vi "calc arcade drive pwm.vi"(3 "error in (no error)":errorcluster, 4 "Y axis value":dbl, 5 "X axis value":dbl) -> (0 "error out":errorcluster, 1 "Right Speed":dbl, 2 "Left Speed":dbl)   [LabVIEW 2013]
uses:
  <vilib>/Rock Robotics/WPI/Solenoid/WPI_SolenoidValue.ctl
  <vilib>/Rock Robotics/SystemInterfaces/NetworkCommunication/NetComm_UsageReport_ResourceType.ctl
  <vilib>/Rock Robotics/WPI/Solenoid/WPI_SolenoidGetEnum.vi
  <vilib>/addons/control/pid/pid.llb/PID (DBL).vi
  <vilib>/Rock Robotics/WPI/RobotDrive/WPI_RobotDriveGetSetRefNum.vi
  <vilib>/addons/control/pid/NI_PID_pid.lvlib
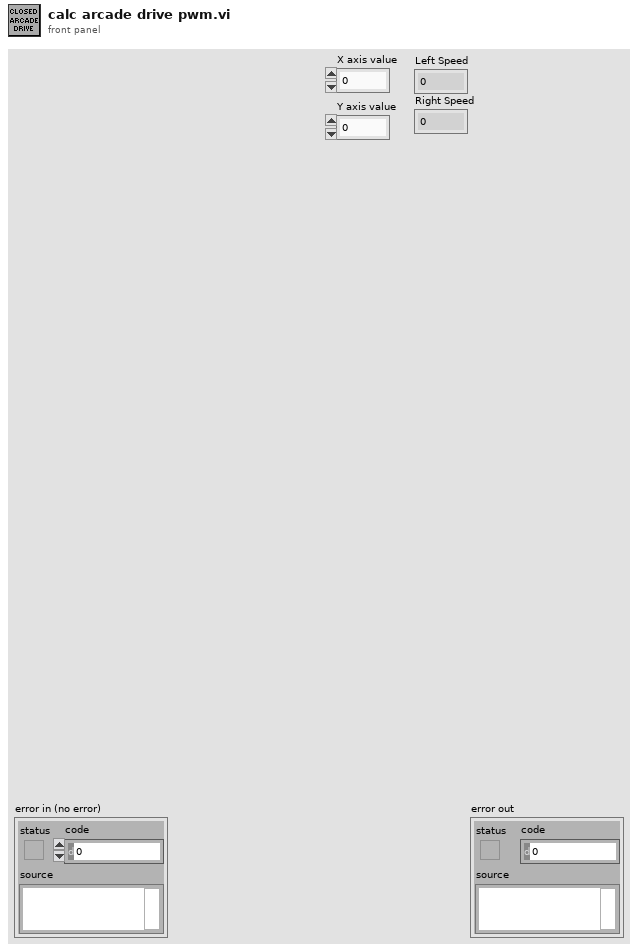
[diagram p1: front panel]
types:
  T1 = cluster{"proportional gain (Kc)":dbl, "integral time (Ti, min)":dbl, "derivative time (Td, min)":dbl}
  T2 = typedef "WPI_SolenoidValue.ctl" = enum16{"Off", "On", "Forward", "Reverse"}
  T3 = typedef "WPI_SolenoidDevRef.ctl" = cluster{"DevStatus":errorcluster, "Solenoid Module":T4, "Forward Solenoid Channel":T5, "Reverse Solenoid Channel":T5}
  T4 = typedef "FPGA_TypedefSolenoidModule.ctl" = enum16{"Solenoid Module 1", "Solenoid Module 2"}
  T5 = typedef "WPI_SolenoidChannel.ctl" = enum8{"Solenoid 1", "Solenoid 2", "Solenoid 3", "Solenoid 4", "Solenoid 5", "Solenoid 6", "Solenoid 7", "Solenoid 8", "Invalid"}
  T6 = typedef "WPI_RobotDriveDevRef.ctl" = cluster{"DevStatus":errorcluster, "Motors[]":T7[], "Square Inputs":bool, "Max Output":dbl, "Isochronous":bool}
  T7 = typedef "WPI_MotorControlDeviceRef.ctl" = cluster{"DeviceStatus":errorcluster, "Type":enum16{"PWM", "CAN"}, "PWM":cluster{"Digital Module":T8, "PWM Channel":T9, "DeadBand":T10}, "CAN":cluster{"Device Number":u8, "Control Mode":T11, "Semaphore":T12, "Max Vout":dbl}, "Invert":bool, "TransformRef":T13, "InvTransformRef":T13}
  T8 = typedef "FPGA_TypedefDigitalModule.ctl" = enum16{"Digital Module 1", "Digital Module 2"}
  T9 = typedef "FPGA_DIOPWMChannel.ctl" = enum8{"PWM 1", "PWM 2", "PWM 3", "PWM 4", "PWM 5", "PWM 6", "PWM 7", "PWM 8", "PWM 9", "PWM 10", "Invalid"}
  T10 = typedef "WPI_PWMDeadband.ctl" = cluster{"Name":string, "maxPositivePwm":i32, "minPositivePwm":i32, "centerPwm":i32, "maxNegativePwm":i32, "minNegativePwm":i32, "angularRange":u16}
  T11 = typedef "WPI_CANJaguar_ControlMode.ctl" = enum8{"Percent VBus", "Current", "Speed", "Position", "Voltage"}
  T12 = typedef "Semaphore RefNum" = refnum<k1>
  T13 = typedef "WPI_PWMTransform_ConPane.ctl" = refnum<vi>
  T14 = typedef "NetComm_UsageReport_ResourceType.ctl" = enum8{"Controller", "Module", "Language", "CANPlugin", "Accelerometer", "ADXL345", "AnalogChannel", "AnalogTrigger", "AnalogTriggerOutput", "CANJaguar", "Compressor", "Counter", "Dashboard", "DigitalInput", "DigitalOutput", "DriverStationCIO", "DriverStationEIO", "DriverStationLCD", "Encoder", "GearTooth", "Gyro", "I2C", "Framework", "Jaguar", "Joystick", "Kinect", "KinectStick", "PIDController", "Preferences", "PWM", "Relay", "RobotDrive", "SerialPort", "Servo", "Solenoid", "SPI", "Task", "Ultrasonic", "Victor", "Button", "Command", "AxisCamera", "PCVideoServer", "SmartDashboard", "Talon", "HiTechnicColorSensor", "HiTechnicAccel", "HiTechnicCompass", "SRF08"}
  T15 = typedef "WPI_EncoderDevRef.ctl" = cluster{"DevStatus":errorcluster, "EncoderIndex":T16, "CounterIndex":T17, "DistancePerCount":dbl, "Decoding Type":T18}
  T16 = typedef "FPGA_EncoderIdx.ctl" = enum8{"Enc 0", "Enc 1", "Enc 2", "Enc 3", "Invalid"}
  T17 = typedef "FPGA_CounterCtrSystemIndex.ctl" = enum8{"Ctr 0", "Ctr 1", "Ctr 2", "Ctr 3", "Ctr 4", "Ctr 5", "Ctr 6", "Ctr 7", "Invalid"}
  T18 = typedef "WPI_EncoderType.ctl" = enum16{"1x", "2x", "4x"}
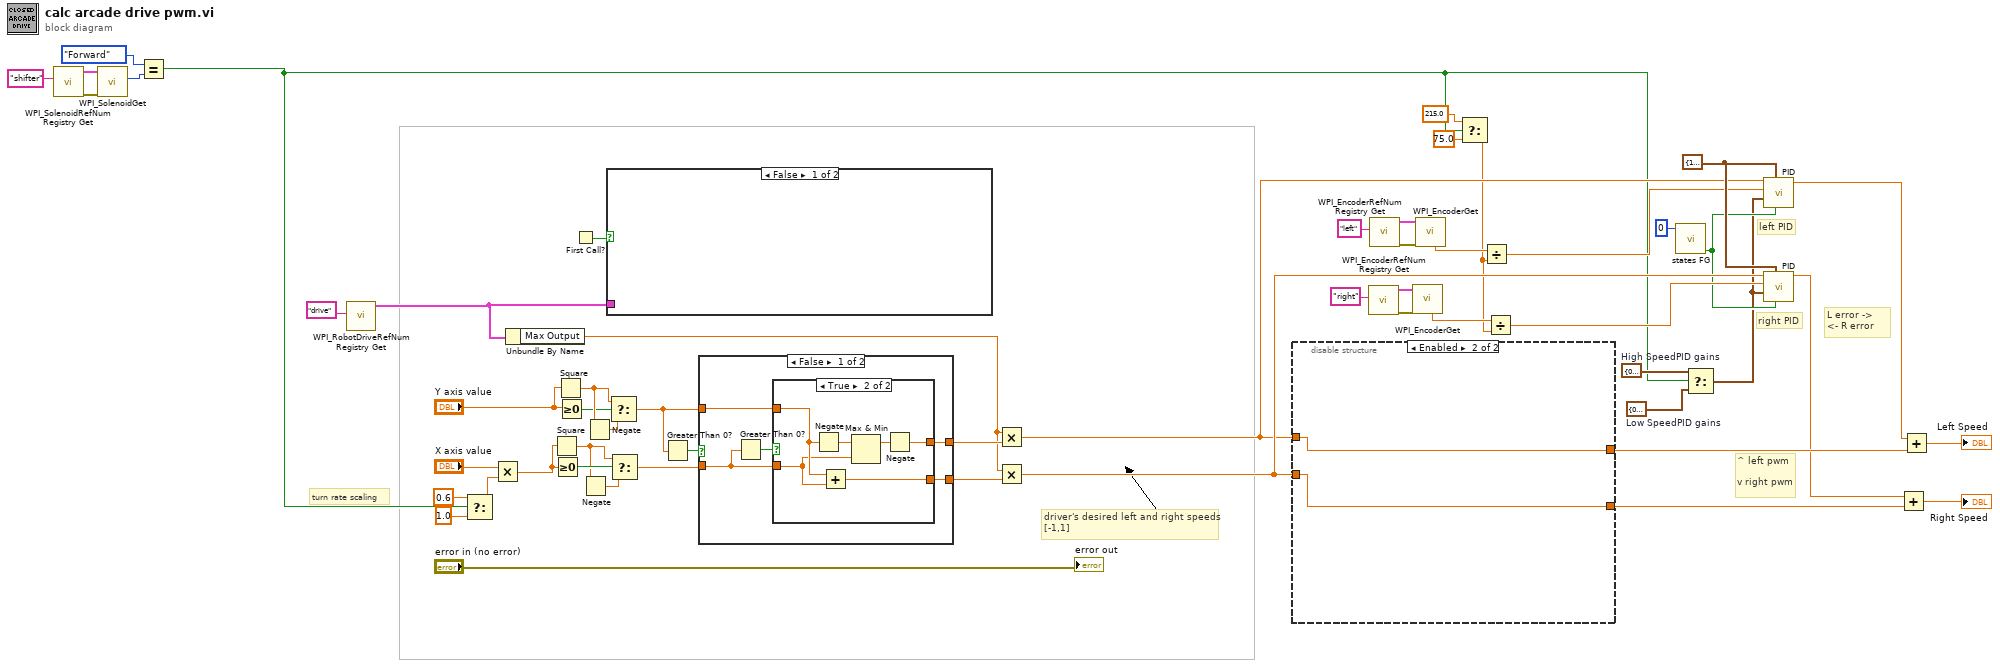
[diagram p0: block diagram]
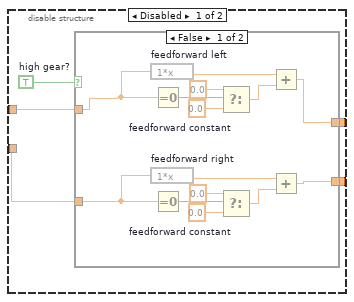
[diagram p2: hidden frame]
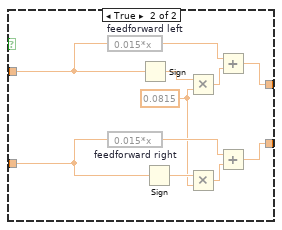
[diagram p3: hidden frame]
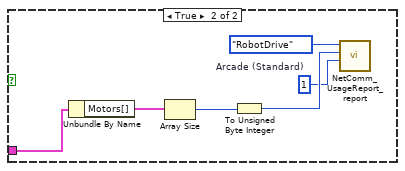
[diagram p4: hidden frame]
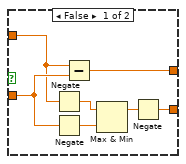
[diagram p5: hidden frame]
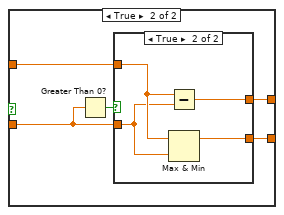
[diagram p6: hidden frame]
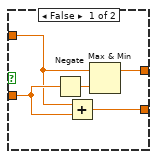
[diagram p7: hidden frame]
diagram:
  w3 = T1 {"proportional gain (Kc)"=0.07, "integral time (Ti, min)"=0.0005, "derivative time (Td, min)"=0.0}  # Low SpeedPID gains
  w4 = T1 {"proportional gain (Kc)"=0.085, "integral time (Ti, min)"=0.0003, "derivative time (Td, min)"=0.0}  # High SpeedPID gains
  w31 = cluster{"output high":dbl, "output low":dbl} {"output high"=1.0, "output low"=-1.0} ("output range")
  # "turn rate scaling"
  # "L error ->\n<- R error"
  # "right PID"
  # "left PID"
  # "^ left pwm\n\nv right pwm"
  # "driver's desired left and right speeds\n[-1,1]"
  n1 = call <vilib>:"WPI_SolenoidRefNum Registry Get.vi"("refnum name"="shifter") -> ("error out"=w18:errorcluster, "SolenoidDevRef"=w17:T3)  [unwired: 9 in]
  n2 = call-poly <vilib>:"WPI_SolenoidGet.vi"("error in (no error)"=w18, "SolenoidDevRef"=w17) -> ("Value"=w16:T2)  [unwired: 7 in, 2 out]
  n3 = Equal?(x=WPI_SolenoidValue."Forward", y=w16) -> (x = y?=w1:bool)
  n4 = call <vilib>:"WPI_RobotDriveRefNum Registry Get.vi"("refnum name"="drive") -> ("RobotDriveDevRef"=w22:T6)  [unwired: 9 in, 1 out]
  n5 = Select(t=0.6, s=w1, f=1.0) -> (s? t:f=w6:dbl)
  n6 = Multiply(x="X axis value", y=w6) -> (x*y=w7:dbl)
  n7 = Unbundle By Name(w22) -> ("Max Output"=w48:dbl)
  n8 = Square(x=w7) -> (x^2=w45:dbl)
  n9 = Greater Or Equal To 0?(x=w7) -> (x >= 0?=w46:bool)
  n10 = Square(x="Y axis value") -> (x^2=w42:dbl)
  n11 = Greater Or Equal To 0?(x="Y axis value") -> (x >= 0?=w41:bool)
  n12 = First Call?() -> (First Call?: T/F=w47:bool)
  n13 = Negate(x=w45) -> (-x=w44:dbl)
  n14 = Negate(x=w42) -> (-x=w43:dbl)
  n15 = case shown="False" w47 {
    tunnel: w22 -> [_ w56]
    frame False {
    }
    frame True {
      w59 = u8 1  # Arcade (Standard)
      n16 = Unbundle By Name(w56) -> ("Motors[]"=w58:T7[])
      n17 = Array Size(array=w58) -> (size(s)=w57:i32)
      n18 = To Unsigned Byte Integer(number=w57) -> (unsigned 8bit integer=w60:u8)
      n19 = call <vilib>:"NetComm_UsageReport_report.vi"("Context"=w59, "Instance Number"=w60, "Resource Type"=NetComm_UsageReport_ResourceType."RobotDrive") -> ()  [unwired: 9 in]
    }
  }
  n20 = Select(t=w42, s=w41, f=w43) -> (s? t:f=w54:dbl)
  n21 = Select(t=w45, s=w46, f=w44) -> (s? t:f=w53:dbl)
  n22 = Greater Than 0?(x=w54) -> (x > 0?=w55:bool)
  n23 = case shown="False" w55 {
    tunnel: w53 -> [w65 w83]
    tunnel: w54 -> [w64 w82]
    tunnel: [w63 w81] -> w52
    tunnel: [w62 w80] -> w49
    frame False {
      n24 = Greater Than 0?(x=w65) -> (x > 0?=w66:bool)
      n25 = case shown="True" w66 {
        tunnel: w65 -> [w73 w75]
        tunnel: w64 -> [w71 w76]
        tunnel: [w67 w77] -> w63
        tunnel: [w68 w74] -> w62
        frame False {
          n26 = Negate(x=w71) -> (-x=w72:dbl)
          n27 = Negate(x=w73) -> (-x=w70:dbl)
          n28 = Subtract(x=w71, y=w73) -> (x-y=w67:dbl)
          n29 = Max & Min(x=w72, y=w70) -> (max(x,y)=w69:dbl)  [unwired: 1 out]
          n30 = Negate(x=w69) -> (-x=w68:dbl)
        }
        frame True {
          n31 = Negate(x=w76) -> (-x=w79:dbl)
          n32 = Add(x=w76, y=w75) -> (x+y=w74:dbl)
          n33 = Max & Min(x=w79, y=w75) -> (max(x,y)=w78:dbl)  [unwired: 1 out]
          n34 = Negate(x=w78) -> (-x=w77:dbl)
        }
      }
    }
    frame True {
      n35 = Greater Than 0?(x=w83) -> (x > 0?=w84:bool)
      n36 = case shown="True" w84 {
        tunnel: w83 -> [w89 w91]
        tunnel: w82 -> [w86 w92]
        tunnel: [w87 w90] -> w81
        tunnel: [w85 w93] -> w80
        frame False {
          n37 = Negate(x=w89) -> (-x=w88:dbl)
          n38 = Add(x=w86, y=w89) -> (x+y=w85:dbl)
          n39 = Max & Min(x=w86, y=w88) -> (max(x,y)=w87:dbl)  [unwired: 1 out]
        }
        frame True {
          n40 = Subtract(x=w92, y=w91) -> (x-y=w90:dbl)
          n41 = Max & Min(x=w92, y=w91) -> (max(x,y)=w93:dbl)  [unwired: 1 out]
        }
      }
    }
  }
  n42 = Multiply(x=w48, y=w52) -> (x*y=w20:dbl)
  n43 = Multiply(x=w48, y=w49) -> (x*y=w21:dbl)
  n44 = disable-structure shown="Enabled" {
    disable-tunnel: [w97 w125] -> w28
    disable-tunnel: [w96 w124] -> w27
    disable-tunnel: w21 -> [w95 w124]
    disable-tunnel: w20 -> [w94 w125]
    frame Disabled {
      w98 = TRUE  # high gear?
      n45 = case shown="False" w98 {
        tunnel: w94 -> [w107 w120]
        tunnel: w95 -> [w101 w115]
        tunnel: [w100 w119] -> w97
        tunnel: [w99 w114] -> w96
        frame False {
          w103 = 0.0  # feedforward constant
          w111 = 0.0  # feedforward constant
          n46 = expression code="1*x" "feedforward left"(w107) -> (w108:dbl)
          n47 = expression code="1*x" "feedforward right"(w101) -> (w106:dbl)
          n48 = Equal To 0?(x=w107) -> (x = 0?=w109:bool)
          n49 = Equal To 0?(x=w101) -> (x = 0?=w105:bool)
          n50 = Select(t=0.0, s=w109, f=w111) -> (s? t:f=w112:dbl)
          n51 = Select(t=0.0, s=w105, f=w103) -> (s? t:f=w102:dbl)
          n52 = Add(x=w108, y=w112) -> (x+y=w100:dbl)
          n53 = Add(x=w106, y=w102) -> (x+y=w99:dbl)
        }
        frame True {
          w113 = 0.0815
          n54 = expression code="0.015*x" "feedforward left"(w120) -> (w121:dbl)
          n55 = expression code="0.015*x" "feedforward right"(w115) -> (w116:dbl)
          n56 = Sign(1:w120) -> (0:w123:dbl)
          n57 = Sign(1:w115) -> (0:w118:dbl)
          n58 = Multiply(x=w123, y=w113) -> (x*y=w122:dbl)
          n59 = Multiply(x=w118, y=w113) -> (x*y=w117:dbl)
          n60 = Add(x=w121, y=w122) -> (x+y=w119:dbl)
          n61 = Add(x=w116, y=w117) -> (x+y=w114:dbl)
        }
      }
    }
    frame Enabled {
    }
  }
  n62 = call <vilib>:"WPI_EncoderRefNum Registry Get.vi"("refnum name"="right") -> ("error out"=w34:errorcluster, "EncoderDevRef"=w35:T15)  [unwired: 9 in]
  n63 = call <vilib>:"WPI_EncoderRefNum Registry Get.vi"("refnum name"="left") -> ("error out"=w37:errorcluster, "EncoderDevRef"=w36:T15)  [unwired: 9 in]
  n64 = call <vilib>:"WPI_EncoderGet.vi"("error in (no error)"=w34, "EncoderDevRef"=w35) -> ("Rate"=w32:dbl)  [unwired: 4 in, 5 out]
  n65 = call <vilib>:"WPI_EncoderGet.vi"("error in (no error)"=w37, "EncoderDevRef"=w36) -> ("Rate"=w33:dbl)  [unwired: 4 in, 5 out]
  n66 = Select(t=215.0, s=w1, f=75.0) -> (s? t:f=w10:dbl)
  n67 = Divide(x=w33, y=w10) -> (x/y=w14:dbl)
  n68 = Divide(x=w32, y=w10) -> (x/y=w13:dbl)
  n69 = call "states FG.vi"("Loop ID"=0) -> ("first call?"=w5:bool)  [unwired: 7 in, 3 out]
  n70 = Select(t=w4, s=w1, f=w3) -> (s? t:f=w2:T1)
  n71 = call-poly <vilib>:"PID.vi"("reinitialize? (F)"=w5, "output range"=w31, "PID gains"=w2, "process variable"=w14, "setpoint"=w20) -> ("output"=w29:dbl)  [unwired: 5 in, 1 out]
  n72 = call-poly <vilib>:"PID.vi"("reinitialize? (F)"=w5, "output range"=w31, "PID gains"=w2, "process variable"=w13, "setpoint"=w21) -> ("output"=w26:dbl)  [unwired: 5 in, 1 out]
  n73 = Add(x=w26, y=w27) -> (x+y=→"Right Speed":dbl)
  n74 = Add(x=w29, y=w28) -> (x+y=→"Left Speed":dbl)
  "error out" <- "error in (no error)"
